vi "Read Data.vi"(8 "error in (no error)":errorcluster, 11 "2D Single Data in":refnum<class "2D Single Data.lvclass">) -> (0 "error out":errorcluster, 2 "Data":sgl[][](array[numeric]), 3 "2D Single Data out":refnum<class "2D Single Data.lvclass">)   [LabVIEW 2012, in "Base Data Class.lvlib" / "2D Single Data.lvclass"]
uses:
  2D Single Data.lvclass
  2D Single Data.lvclass/2D Single Data.ctl
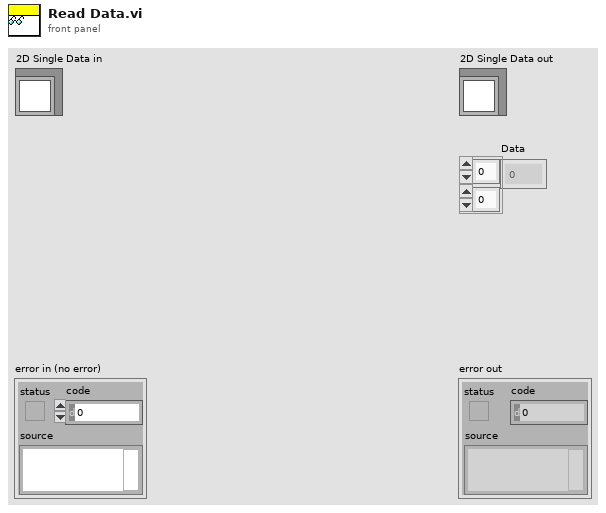
[diagram p1: front panel]
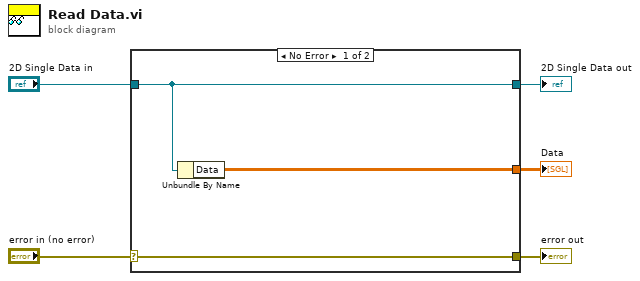
[diagram p0: block diagram]
diagram:
  n1 = case shown="No Error" "error in (no error)" {
    selector: "error in (no error)" -> [w8 w9]
    tunnel: [w8 w9] -> w4
    tunnel: [w7 w10] -> w2
    tunnel: "2D Single Data in" -> [w7 w10]
    tunnel: [w6 _] -> w1
    frame No Error {
      n2 = Unbundle By Name(w7) -> ("Data"=w6:sgl[][])
    }
    frame Error {
    }
  }
  "error out" <- w4
  "2D Single Data out" <- w2
  "Data" <- w1
